vi "tb_Acquire Data from Single Channel.vi"() -> ()   [LabVIEW 2012]
uses:
  Acquisition Engine/Acquisition Engine State.ctl
  <vilib>/Platform/TimedLoop/XDataNode/timing_clust.ctl
  <vilib>/Platform/TimedLoop/XDataNode/nitl_modes.ctl
  <vilib>/Platform/TimedLoop/XDataNode/wakeup.ctl
  <vilib>/rvi/Emulation/niFpgaSctlEmulationRegisterWithScheduler.vi
  <vilib>/rvi/Emulation/niFpgaSctlEmulationScheduler.vi
  <vilib>/rvi/interface/RandomDataEmulation/nirviRandomDataFPGAFIFO.vi
  <vilib>/rvi/interface/RandomDataEmulation/niFpgaRandomDataHandleErrors.vi
  <vilib>/Platform/TimedLoop/XDataNode/XDataNode.xnode
  <vilib>/rvi/DataTransferAndStorage/Container/XNode/niFpgaContainer.xnode
  <vilib>/rvi/interface/RandomDataEmulation/nirviRandomDataFpgaReadWriteTemplate.vi
  <vilib>/Platform/TimedLoop/XDataNode/XDNodeRunTimeDep.lvlib
panel:
  out "Host Inputs":T1
  in  "Record Count":u16=1
  in  "Trigger Hold Off":u16
  in  "Load Record Parameters?":bool
  in  "Samples per Record":u16=1000
  in  "Pre Trigger Samples":u16
  out "Data Acquired":i16(graph)
  in  "Trigger Type":T2(ring)=enum."Software Trigger"
  out "Current State":T3=enum."Arm Acquisition Engine"
  out "Points Acquired":u64
  out "Host FIFO Time Out":bool
  in  "Channel":T4(ring)
  in  "Software Trigger from Host":bool
  in  "Arm Acquisition Engine":bool
  in  "Reset?":bool
  # "Points Acquired = Samples per Record + 1"
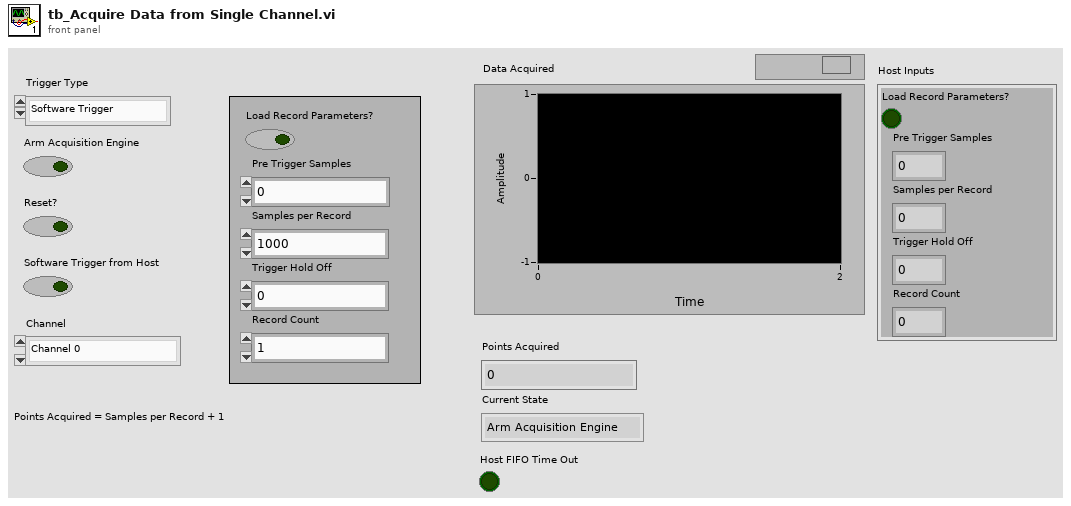
[diagram p1: front panel]
types:
  T1 = cluster{"Load Record Parameters?":bool, "Pre Trigger Samples":u16, "Samples per Record":u16, "Trigger Hold Off":u16, "Record Count":u16}
  T2 = enum8{"External Digital Trigger", "Software Trigger", "Immediate Trigger"}
  T3 = typedef "Acquisition Engine State.ctl" = enum8{"Idle", "Arm Acquisition Engine", "Acquire Pre-Trigger Samples", "Wait for Trigger", "Acquisition Hold Off Time", "Read Data from Buffer", "Check Records Done?", "Re-Arm State", "Flush Available Data"}
  T4 = enum16{"Channel 0", "Channel 1", "Channel 2", "Channel 3"}
  T5 = typedef "XDNodeRunTimeDep.lvlib/timing_clust.ctl" = cluster{"Expected End [f-1]":u64, "Actual End [f-1]":u64, "Finished Late? [f-1]":bool, "Expected End [i-1]":u64, "Actual End [i-1]":u64, "Finished Late? [i-1]":bool, "Expected Start [i]":u64, "Actual Start [i]":u64, "Expected Start [f]":u64, "Actual Start [f]":u64, "Source Name":string, "Structure Name":string, "Period":i64, "Deadline":i64, "Offset":i64, "Start":i64, "Priority":i32, "Timeout":i32, "Mode":T6, "Wakeup Reason":T7, "Error":errorcluster, "Source Type":string, "Secondary Source Type":string, "Global End Time":u64, "Global Start Time":u64, "Frame Duration":u64, "Iteration Duration":u64, "Assigned CPU":i32, "I/O Scan Engine Mode":u32}
  T6 = typedef "XDNodeRunTimeDep.lvlib/nitl_modes.ctl" = enum32{"No Change", "Process missed periods, maintain original phase", "Discard missed periods, maintain original phase", "Process missed periods, ignore original phase", "Discard missed periods, ignore original phase"}
  T7 = typedef "XDNodeRunTimeDep.lvlib/wakeup.ctl" = enum32{"Normal", "Aborted", "Asynchronous wakeup", "Timing source error", "Timed loop error", "Timeout"}
  T8 = typedef "Multi-Channel Analog Input Data.ctl" = i16[]
  T9 = typedef "Acquisition Parameters.ctl" = cluster{"Pre Trigger Samples":u16, "Post-Trigger Samples":u16, "Trigger Hold Off":u16, "Record Count":u16}
  T10 = typedef "Buffer Parameters.ctl" = cluster{"Init Read and Write Pointer":bool, "Write Pointer":u16, "Read Pointer":u16, "Buffer Length-1":u16}
  T11 = typedef "Acquisition Status.ctl" = cluster{"Reset":bool, "Acquisition Engine Start (Arm)":bool, "Current State":T3, "Trig Offset":u8, "Points Unread":u16, "Points Acquired":u16, "Records Done":u16, "Start of Read":bool, "End of Read":bool, "Start of Record":bool, "End of Record":bool, "Ready for Ref Trig":bool, "In Reset?":bool}
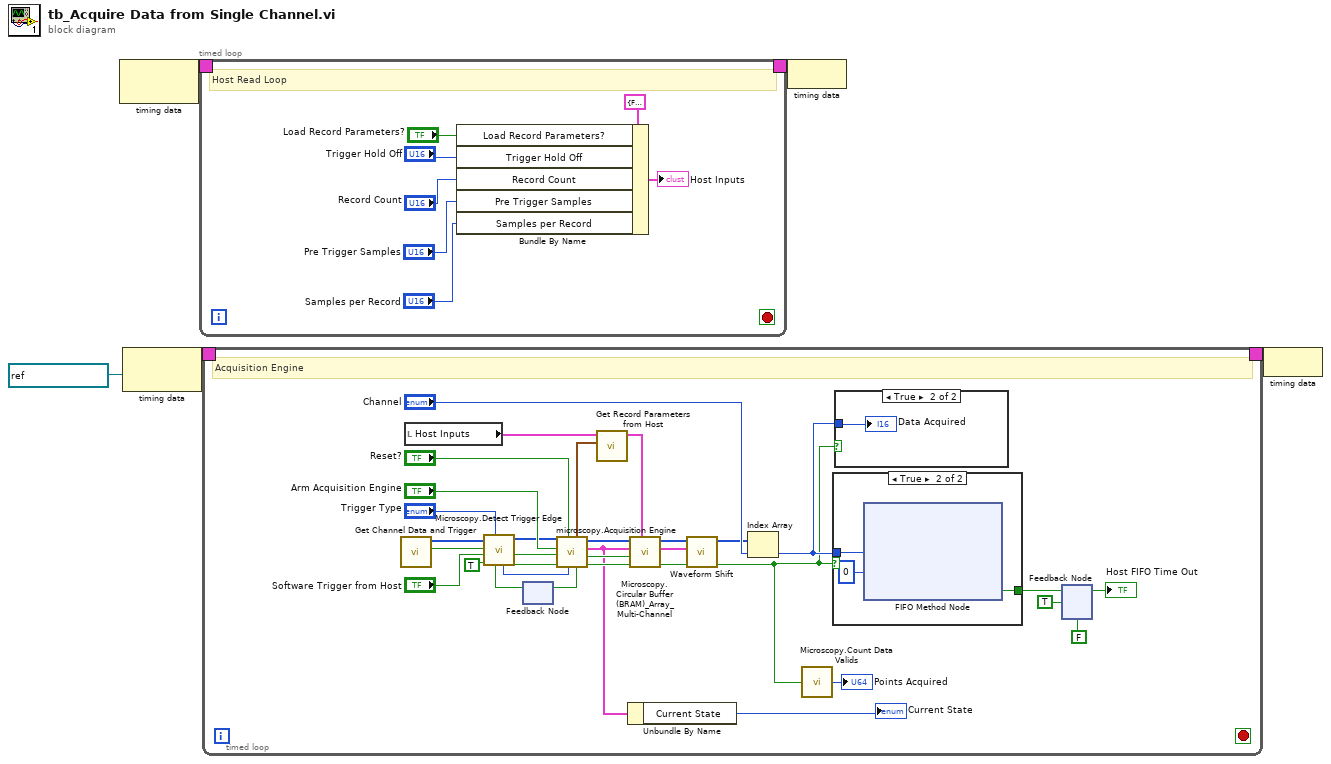
[diagram p0: block diagram]
diagram:
  n1 = node-c288() -> (w2:T5)  [unwired: 1 in]
  n2 = node-c288(refnum<k21> "ADC Clock" ("Source Name")) -> (w5:T5)
  n3 = timed-loop {
    timing: w2 -> [_]
    timing-out: [_] -> w1
    stop <- _ stop-if-true
    # "Host Read Loop"
    n4 = Bundle By Name(cluster=T1 {"Load Record Parameters?"=FALSE, "Pre Trigger Samples"=0, "Samples per Record"=0, "Trigger Hold Off"=0, "Record Count"=0} ("Record Parameters"), "Load Record Parameters?"="Load Record Parameters?", "Trigger Hold Off"="Trigger Hold Off", "Record Count"="Record Count", "Pre Trigger Samples"="Pre Trigger Samples", "Samples per Record"="Samples per Record") -> (→"Host Inputs":T1)
  }
  n5 = timed-loop {
    timing: w5 -> [_]
    timing-out: [_] -> w4
    stop <- _ stop-if-true
    # "Acquisition Engine"
    n6 = call "Get Channel Data and Trigger.vi"() -> ("Trigger"=w24:bool, "Data"=w34:i16[])  [unwired: 10 in]
    n7 = local read "Host Inputs"() -> (w21:T1)
    n8 = feedback #1() -> (w27:bool)  [unwired: 1 in]
    n9 = call "Microscopy.Detect Trigger Edge.vi"("Ready for Next Record?"=w27, "Trigger Type"="Trigger Type", "Data Valid In"=TRUE, "Software Trigger from Host"="Software Trigger from Host", "Digita IO Trigger"=w24, "Analog Channel Data"=w34) -> ("Data Valid Out"=w40:bool, "Reference Trigger Edge?"=w41:bool, "Analog Channel Data"=w42:T8, "Trig Offset"=w15:u8)  [unwired: 2 in]
    n10 = call "Get Record Parameters from Host.vi"("Record Parameters"=w21) -> ("Acquisition Parameters"=w37:T9, "Buffer Parameters"=w36:T10)  [unwired: 9 in]
    n11 = call "microscopy.Acquisition Engine.vi"("Acquisition Parameters"=w37, "Trig Offset"=w15, "Reset?"="Reset?", "Data Valid In"=w40, "Reference Trigger Edge?"=w41, "Arm Acquisition Engine"="Arm Acquisition Engine", "Channel Data In"=w42) -> ("Data Valid Out"=w43:bool, "Read from Buffer"=w44:bool, "Acquisition Status"=w26:T11, "Channel Data Out"=w45:T8, "Ready for Ref Trig"=w28:bool)
    n12 = feedback-in #1(w28) -> ()
    n13 = Unbundle By Name(w26) -> ("Current State"=→"Current State":T3)
    n14 = call "Microscopy.Circular Buffer (BRAM)_Array_Multi-Channel.vi"("Buffer Pointers"=w36, "Input Valid"=w43, "Read Data?"=w44, "Acquisition Status In"=w26, "Input Write Data"=w45) -> ("Output Valid"=w17:bool, "Acquisition Status Out"=w19:T11, "Output Write Data"=w20:T8)  [unwired: 4 in]
    n15 = call "Waveform Shift.vi"("Input Data Valid"=w17, "Acquisition Status In"=w19, "Input Data"=w20) -> ("Output Data Valid"=w16:bool, "Output Data"=w18:i16[])  [unwired: 6 in, 1 out]
    n16 = Index Array(array=w18, index="Channel") -> (element=w22:i16)
    n17 = call "Microscopy.Count Data Valids.vi"("Data Valid"=w16) -> ("Counter"=→"Points Acquired":u64)  [unwired: 14 in]
    n18 = case shown="True" w16 {
      tunnel: w22 -> [_ w51]
      tunnel: [_ w49] -> w33
      frame False {
      }
      frame True {
        n19 = xnode ("FIFO Method Node")("Element"=w51, "Timeout"=0) -> ("Timed Out?"=w49:bool)  [unwired: 1 in, 1 out]
      }
    }
    n20 = case shown="True" w16 {
      tunnel: w22 -> [_ w48]
      frame False {
      }
      frame True {
        "Data Acquired" <- w48
      }
    }
    n21 = feedback-in #2(w33, TRUE) -> ()
    n22 = feedback #2(FALSE ("Timed Out?")) -> (→"Host FIFO Time Out":bool)
  }
  n23 = node-c288(w1) -> ()
  n24 = node-c288(w4) -> ()
